vi "WPI_SolenoidSafetyTest.vi"   [LabVIEW 2017]
doc: "Calls the SafetyCheck VI. SafetyCheck VI needs to be called dynamically by the SafetyCheckEngine, but it already gets called statically. Wrapping it in this VI enables calling it dynamically."
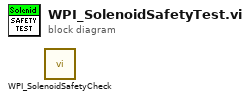
[diagram p0: block diagram]
diagram:
  n1 = call <vilib>:"WPI_SolenoidSafetyCheck.vi"() -> ()  [unwired: 3 in, 13 out]
